vi "Hardware In - ECS - EPTx Interface.vi"(0 "FPGA 1 Ref":T2, 5 "FPGA 2 Ref":T2, 11 "FPGA Knock Ref":T2) -> (4 "EPT out":T3, 6 "Aux1Adv":sgl, 8 "Aux2Adv":sgl, 10 "Aux3Adv":sgl, 12 "Engine Status":T1, 13 "Knock.Intensity":sgl[](array[numeric]) format="%.6g", 14 "Knock.Results":bool[](array[boolean]), 15 "Aux4Adv":sgl)   [LabVIEW 2015, in "ECS-RT.lvlib"]
uses:
  ECS-RT.lvlib
  Typedefs/EPT/EPT Cluster.ctl
  <vilib>/Powertrain Controls/Device Drivers/Engine Position Tracking/EPTx/RevA/RT/Controls/EPTxData.ctl
  Typedefs/FPGA Refs/Generic FPGA Ref.ctl
  Typedefs/EPT/Engine Status.ctl
  <vilib>/Powertrain Controls/Device Drivers/Engine Position Tracking/EPTx/RevA/RT/Controls/EPTxState.ctl
  <vilib>/Powertrain Controls/Device Drivers/Engine Position Tracking/EPTx/RevA/RT/Controls/EPTxFilters.ctl
  <vilib>/Powertrain Controls/Device Drivers/Engine Position Tracking/EPTx/RevA/RT/Controls/Encoder Config.ctl
  <vilib>/Powertrain Controls/Device Drivers/FPGA Knock/RevA/RT/Controls/Knock Settings.ctl
  <vilib>/Powertrain Controls/Device Drivers/FPGA Knock/RevA/RT/Controls/Windows.ctl
  <vilib>/Utility/error.llb/Error Cluster From Error Code.vi
  <vilib>/rvi/errors/niLvFpgaAdjustHostInterfaceError.vi
  Globals/TDC Globals.vi
  <vilib>/rvi/interface/nirviReadWriteControl/nirviReadWriteControl.xnode
  NiFpgaLv.dll
  <vilib>/rvi/interface/Simulation/niFpgaSimulationCallBeginRW.vi
  ECS-Shared.lvlib
  <vilib>/Powertrain Controls/Device Drivers/Engine Position Tracking/EPTx/RevA/RT/EPTx - RevA - RT.lvlib
  <vilib>/Powertrain Controls/Device Drivers/FPGA Knock/RevA/RT/Knock - RevA - RT.lvlib
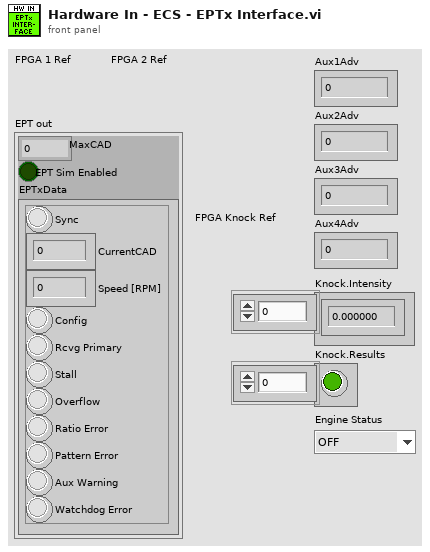
[diagram p1: front panel]
types:
  T1 = typedef "ECS-Shared.lvlib/Engine Status.ctl" = enum16{"OFF", "STALLED", "CRANKING", "RUNNING", "ACCEL", "DECEL", "SAFE"}
  T2 = typedef "ECS-Shared.lvlib/Generic FPGA Ref.ctl" = refnum<k20>
  T3 = typedef "ECS-Shared.lvlib/EPT Cluster.ctl" = cluster{"MaxCAD":sgl, "EPT Sim Enabled":bool, "EPTxData":T4}
  T4 = typedef "EPTx - RevA - RT.lvlib/EPTxData.ctl" = cluster{"Sync":bool, "CurrentCAD":sgl, "Speed [RPM]":sgl, "Config":bool, "Rcvg Primary":bool, "Stall":bool, "Overflow":bool, "Ratio Error":bool, "Pattern Error":bool, "Aux Warning":bool, "Watchdog Error":bool}
  T5 = enum8{"1 Sample/Pulse", "2 Sample/Pulse", "4 Sample/Pulse"}
  T6 = typedef "EPTx - RevA - RT.lvlib/Encoder Config.ctl" = cluster{"Tooth Count":u16, "Max Rate [Hz]":sgl, "Samples":enum8{"1 Sample/Pulse", "2 Sample/Pulse", "4 Sample/Pulse"}}
  T7 = typedef "EPTx - RevA - RT.lvlib/EPTxFilters.ctl" = cluster{"Primary [s]":sgl, "Aux 1 [s]":sgl, "Aux 2 [s]":sgl, "Aux 3 [s]":sgl, "Aux 4 [s]":sgl}
  T8 = typedef "EPTx - RevA - RT.lvlib/EPTxState.ctl" = cluster{"Sync Enable":bool, "Clear Errors":bool, "Sim Enable":bool, "Sim Speed [RPM]":sgl}
  T9 = typedef "Knock - RevA - RT.lvlib/Windows.ctl" = cluster{"Knock Start [CAD]":sgl, "Knock End [CAD]":sgl, "Reference End [CAD]":sgl, "Reference Start [CAD]":sgl}
  T10 = typedef "Knock - RevA - RT.lvlib/Knock Settings.ctl" = cluster{"Frequency [Hz]":sgl, "Low Cutoff [Hz]":sgl, "High Cutoff [Hz]":sgl, "Threshold":sgl}
  T11 = cluster{"Enable":bool, "RisingCAD":fxp<+,18,11>, "FallingCAD":fxp<+,18,11>}
  T12 = cluster{"Sync":bool, "CurrentCAD":fxp<+,18,11>, "MaxCAD":fxp<+,11,11>, "HistoryCAD":fxp<+,11,11>, "CADRate":fxp<+,22,8>, "AvgSpeed":fxp<+,17,15>, "Config":bool, "Rcvg Primary":bool, "Stall":bool, "Overflow":bool, "Ratio Error":bool, "Pattern Error":bool, "Aux Warning":bool, "Watchdog Error":bool}
  T13 = typedef "EPTx - RevA - RT.lvlib/EPTxSettings.ctl" = cluster{"Rotation":u8, "Ratios":sgl[], "Thresholds":sgl[], "Tooth":T14, "Pattern":T16[], "Token":T17[], "Aux Threshold Min":T20, "Aux Threshold Max":T20}
  T14 = typedef "EPTx - RevA - RT.lvlib/Settings - Tooth.ctl" = cluster{"Rising Edge":bool, "Falling Edge":bool, "Direction\nDetection":T15, "Level":bool, "Parameter":sgl}
  T15 = typedef "EPTx - RevA - RT.lvlib/Direction Detection.ctl" = enum16{"None", "Aux Signal", "Length"}
  T16 = typedef "EPTx - RevA - RT.lvlib/Settings - Pattern.ctl" = cluster{"Ratio Index":u8, "Ratio Count":u16, "Angle":sgl, "dAngle":sgl}
  T17 = typedef "EPTx - RevA - RT.lvlib/Settings - Token.ctl" = cluster{"Length":u16, "Start Index":u8, "Start Count":u16, "Aux 1":T18, "Aux 1 Type":T19, "Aux 1 Max":u16, "Aux 1 Min":u16, "Aux 2":T18, "Aux 2 Type":T19, "Aux 2 Max":u16, "Aux 2 Min":u16, "End Index":u8, "End Count":u16}
  T18 = typedef "EPTx - RevA - RT.lvlib/Aux Signal.ctl" = enum8{"---", "Aux 1", "Aux 2", "Aux 3", "Aux 4"}
  T19 = typedef "EPTx - RevA - RT.lvlib/Aux Type.ctl" = enum8{"Falling", "Rising", "Low", "High", "Ratio"}
  T20 = typedef "EPTx - RevA - RT.lvlib/Aux Threshold.ctl" = cluster{"Aux 1":sgl, "Aux 2":sgl, "Aux 3":sgl, "Aux 4":sgl}
  T21 = typedef "EPTx - RevA - FPGA.lvlib/EPTxConfig.ctl" = u64
  T22 = typedef "EPTx - RevA - FPGA.lvlib/EPTxControl.ctl" = cluster{"Sync Enable":bool, "Clear Errors":bool, "Sim Enable":bool, "Sim Rate":fxp<+,24,6>, "Watchdog":bool}
  T23 = typedef "Knock - RevA - FPGA.lvlib/Knock Settings.ctl" = cluster{"Threshold":fxp<+,8,4>, "Coeff A":fxp<+/-,16,4>[], "Coeff B":fxp<+/-,16,4>[]}
  T24 = typedef "Knock - RevA - FPGA.lvlib/EPTx Window.ctl" = cluster{"Knock Start":fxp<+,18,11>, "Knock End":fxp<+,18,11>, "Reference Start":fxp<+,18,11>, "Reference End":fxp<+,18,11>}
  T25 = typedef "EPTx - RevA - FPGA.lvlib/EPTxEncoderConfig.ctl" = cluster{"Tooth Count":fxp<+,12,12>, "Rate Limit":fxp<+,12,12>}
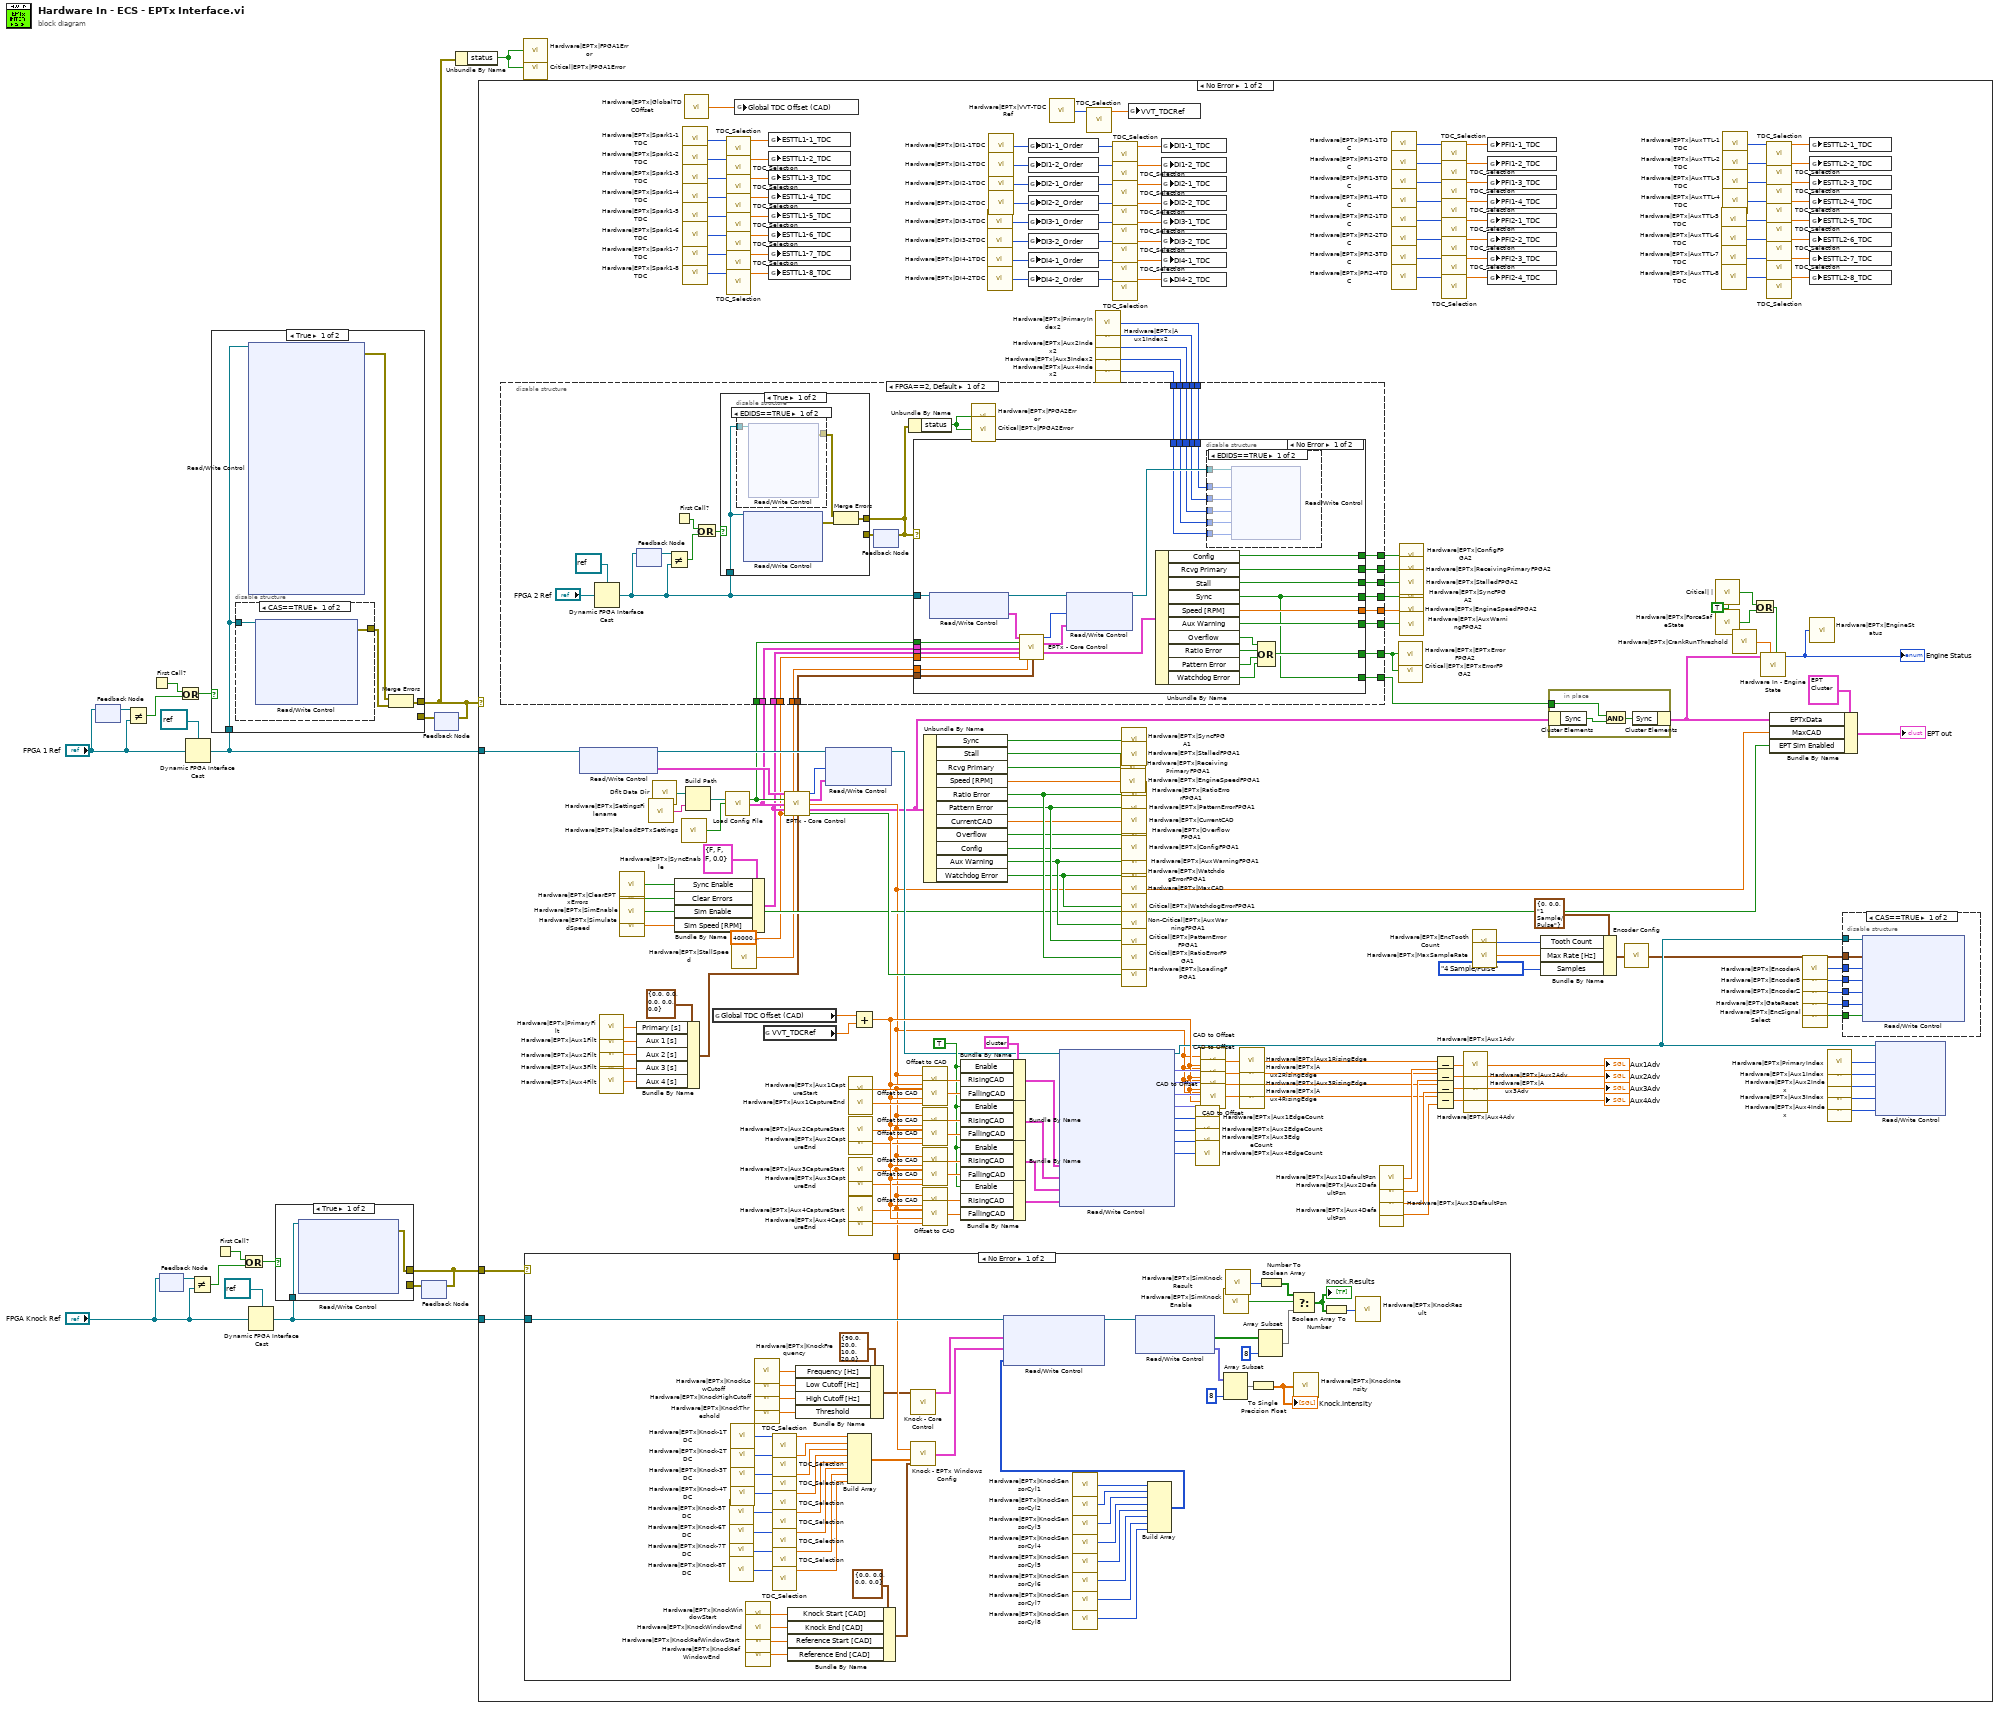
[diagram p0: block diagram]
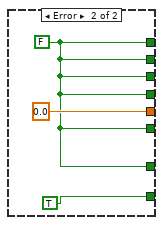
[diagram p6: hidden frame]
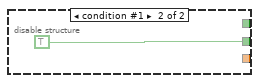
[diagram p9: hidden frame]
diagram:
  n1 = feedback #1() -> (w18:T2)  [unwired: 1 in]
  n2 = feedback-in #1("FPGA 1 Ref") -> ()
  n3 = Not Equal?(x=w18, y="FPGA 1 Ref") -> (x != y?=w19:bool)
  n4 = First Call?() -> (First Call?: T/F=w17:bool)
  n5 = feedback #2() -> (w8:T2)  [unwired: 1 in]
  n6 = feedback-in #2("FPGA Knock Ref") -> ()
  n7 = Or(x=w17, y=w19) -> (x .or. y?=w16:bool)
  n8 = Dynamic FPGA Interface Cast(Session In=refnum<k20> refnum ("EPT"), Type="FPGA 1 Ref") -> (Session Out=w12:refnum<k20>)
  n9 = Not Equal?(x=w8, y="FPGA Knock Ref") -> (x != y?=w9:bool)
  n10 = First Call?() -> (First Call?: T/F=w7:bool)
  n11 = Or(x=w7, y=w9) -> (x .or. y?=w6:bool)
  n12 = Dynamic FPGA Interface Cast(Session In=refnum<k20> refnum ("EPT"), Type="FPGA Knock Ref") -> (Session Out=w2:refnum<k20>)
  n13 = feedback #3() -> (w5:errorcluster)  [unwired: 1 in]
  n14 = case shown="True" w6 {
    tunnel: [w20 w22] -> w3
    tunnel: w5 -> [_ w22]
    tunnel: w2 -> [w21 _]
    frame True {
      n15 = xnode "Read/Write Control"("FPGA VI Reference In"=w21) -> ("error out"=w20:errorcluster)  [unwired: 4 in, 3 out]
    }
    frame False {
    }
  }
  n16 = feedback-in #3(w3) -> ()
  n17 = feedback #4() -> (w15:errorcluster)  [unwired: 1 in]
  n18 = case shown="True" w16 {
    tunnel: [w25 w29] -> w11
    tunnel: w15 -> [_ w29]
    tunnel: w12 -> [w26 _]
    frame True {
      n19 = disable-structure shown="CAS==TRUE" {
        disable-tunnel: w26 -> [w28 _]
        disable-tunnel: [w27 _] -> w23
        frame condition #0 (active) {
          n20 = xnode "Read/Write Control"("FPGA VI Reference In"=w28) -> ("error out"=w27:errorcluster)  [unwired: 7 in, 1 out]
        }
        frame condition #1 {
        }
      }
      n21 = xnode "Read/Write Control"("FPGA VI Reference In"=w26) -> ("error out"=w24:errorcluster)  [unwired: 12 in, 10 out]
      n22 = Merge Errors(w24, w23) -> (w25:errorcluster)
    }
    frame False {
    }
  }
  n23 = feedback-in #4(w11) -> ()
  n24 = Unbundle By Name(w11) -> ("status"=w10:bool)
  n25 = case shown="No Error" w11 {
    tunnel: w12 -> [w120 _]
    tunnel: w3 -> [w90 _]
    tunnel: w2 -> [w89 _]
    frame No Error {
      w109 = sgl 40000000.0 ("Frequency (40M) [Hz]")
      w125 = TRUE ("Enable")
      w147 = T11 {"Enable"=FALSE, "RisingCAD"=0.0, "FallingCAD"=0.0} ("EPTx.Aux1AngleCapture")
      n26 = xnode "Read/Write Control"("FPGA VI Reference In"=w120) -> ("FPGA VI Reference Out"=w190:refnum<k20>, "EPTxSupervisor"=w205:T12)  [unwired: 1 in, 1 out]
      n27 = call "Hardware|EPTx|PrimaryFilt"() -> ("Value"=w117:sgl)
      n28 = call "Hardware|EPTx|Aux1Filt"() -> ("Value"=w116:sgl)
      n29 = call "Hardware|EPTx|Aux2Filt"() -> ("Value"=w115:sgl)
      n30 = call "Hardware|EPTx|Aux3Filt"() -> ("Value"=w114:sgl)
      n31 = call "Hardware|EPTx|Aux4Filt"() -> ("Value"=w113:sgl)
      n32 = call "Hardware|EPTx|SyncEnable"() -> ("Value"=w122:bool)
      n33 = call "Hardware|EPTx|ClearEPTxErrors"() -> ("Value"=w101:bool)
      n34 = call "Hardware|EPTx|SimEnable"() -> ("Value"=w119:bool)
      n35 = call "Hardware|EPTx|SimulatedSpeed"() -> ("Value"=w121:sgl)
      n36 = Bundle By Name(cluster=T7 {"Primary [s]"=0.0, "Aux 1 [s]"=0.0, "Aux 2 [s]"=0.0, "Aux 3 [s]"=0.0, "Aux 4 [s]"=0.0} ("Filters (0)"), "Primary [s]"=w117, "Aux 1 [s]"=w116, "Aux 2 [s]"=w115, "Aux 3 [s]"=w114, "Aux 4 [s]"=w113) -> (w108:T7)
      n37 = call "Hardware|EPTx|SettingsFilename"() -> ("Value"=w186:string)
      n38 = call <vilib>:"Dflt Data Dir.vi"() -> ("App:Default Data Directory"=w187:path)
      n39 = Bundle By Name(cluster=T8 {"Sync Enable"=FALSE, "Clear Errors"=FALSE, "Sim Enable"=FALSE, "Sim Speed [RPM]"=0.0} ("EPTxState"), "Sync Enable"=w122, "Clear Errors"=w101, "Sim Enable"=w119, "Sim Speed [RPM]"=w121) -> (w110:T8)
      n40 = call "Hardware|EPTx|ReloadEPTxSettings"() -> ("Value"=w184:bool)
      n41 = call "Hardware|EPTx|Spark1-1TDC"() -> ("Value"=w76:u32)
      n42 = call "Hardware|EPTx|Spark1-2TDC"() -> ("Value"=w75:u32)
      n43 = call "Hardware|EPTx|Spark1-3TDC"() -> ("Value"=w74:u32)
      n44 = call "Hardware|EPTx|Spark1-4TDC"() -> ("Value"=w73:u32)
      n45 = call "Hardware|EPTx|Spark1-5TDC"() -> ("Value"=w72:u32)
      n46 = call "Hardware|EPTx|Spark1-6TDC"() -> ("Value"=w71:u32)
      n47 = call "Hardware|EPTx|Spark1-7TDC"() -> ("Value"=w70:u32)
      n48 = call "Hardware|EPTx|Spark1-8TDC"() -> ("Value"=w69:u32)
      n49 = call "Hardware|EPTx|GlobalTDCOffset"() -> ("Value"=w148:sgl)
      n50 = Build Path(base path=w187, name or relative path=w186) -> (appended path=w185:path)
      n51 = global read "TDC Globals.vi" "Global TDC Offset (CAD)"() -> (w214:sgl)
      n52 = call <vilib>:"Load Config File.vi"("Configuration Path"=w185, "Load"=w184) -> ("Loaded"=w112:bool, "EPTxSettings"=w111:T13)  [unwired: 12 in]
      n53 = call "TDC_Selection.vi"("TDC#"=w76) -> ("TDC"=w183:sgl)  [unwired: 10 in]
      n54 = call "TDC_Selection.vi"("TDC#"=w75) -> ("TDC"=w176:sgl)  [unwired: 10 in]
      n55 = call "TDC_Selection.vi"("TDC#"=w74) -> ("TDC"=w177:sgl)  [unwired: 10 in]
      n56 = call "TDC_Selection.vi"("TDC#"=w73) -> ("TDC"=w178:sgl)  [unwired: 10 in]
      n57 = call "TDC_Selection.vi"("TDC#"=w72) -> ("TDC"=w179:sgl)  [unwired: 10 in]
      n58 = call "TDC_Selection.vi"("TDC#"=w71) -> ("TDC"=w180:sgl)  [unwired: 10 in]
      n59 = call "TDC_Selection.vi"("TDC#"=w70) -> ("TDC"=w181:sgl)  [unwired: 10 in]
      n60 = call "TDC_Selection.vi"("TDC#"=w69) -> ("TDC"=w182:sgl)  [unwired: 10 in]
      n61 = call "Hardware|EPTx|StallSpeed"() -> ("Value"=w91:sgl)
      n62 = global write "TDC Globals.vi" "Global TDC Offset (CAD)"(w148) -> ()
      n63 = global read "TDC Globals.vi" "VVT_TDCRef"() -> (w99:sgl)
      n64 = global write "TDC Globals.vi" "ESTTL1-1_TDC"(w183) -> ()
      n65 = global write "TDC Globals.vi" "ESTTL1-2_TDC"(w176) -> ()
      n66 = global write "TDC Globals.vi" "ESTTL1-3_TDC"(w177) -> ()
      n67 = global write "TDC Globals.vi" "ESTTL1-4_TDC"(w178) -> ()
      n68 = global write "TDC Globals.vi" "ESTTL1-5_TDC"(w179) -> ()
      n69 = global write "TDC Globals.vi" "ESTTL1-6_TDC"(w180) -> ()
      n70 = global write "TDC Globals.vi" "ESTTL1-7_TDC"(w181) -> ()
      n71 = global write "TDC Globals.vi" "ESTTL1-8_TDC"(w182) -> ()
      n72 = call <vilib>:"EPTx - Core Control.vi"("EPTxSupervisor"=w205, "Load"=w112, "EPTxSettings"=w111, "EPTxState"=w110, "Frequency (40M) [Hz]"=w109, "Stall Speed (200) [RPM]"=w91, "Filters (0)"=w108) -> ("EPTxConfig"=w189:T21, "EPTxControl"=w188:T22, "Max CAD"=w88:sgl, "EPTxData"=w87:T4, "Loading"=w195:bool)  [unwired: 4 in]
      n73 = case shown="No Error" w90 {
        tunnel: w89 -> [w254 _]
        tunnel: w88 -> [w233 _]
        frame No Error {
          n74 = call "Hardware|EPTx|Knock-5TDC"() -> ("Value"=w267:u32)
          n75 = call "Hardware|EPTx|Knock-6TDC"() -> ("Value"=w266:u32)
          n76 = call "Hardware|EPTx|Knock-7TDC"() -> ("Value"=w265:u32)
          n77 = call "Hardware|EPTx|Knock-8TDC"() -> ("Value"=w264:u32)
          n78 = call "Hardware|EPTx|Knock-1TDC"() -> ("Value"=w271:u32)
          n79 = call "Hardware|EPTx|Knock-2TDC"() -> ("Value"=w270:u32)
          n80 = call "Hardware|EPTx|Knock-3TDC"() -> ("Value"=w269:u32)
          n81 = call "Hardware|EPTx|Knock-4TDC"() -> ("Value"=w268:u32)
          n82 = call "Hardware|EPTx|KnockWindowStart"() -> ("Value"=w275:sgl)
          n83 = call "Hardware|EPTx|KnockWindowEnd"() -> ("Value"=w274:sgl)
          n84 = call "Hardware|EPTx|KnockRefWindowStart"() -> ("Value"=w273:sgl)
          n85 = call "Hardware|EPTx|KnockRefWindowEnd"() -> ("Value"=w272:sgl)
          n86 = call "Hardware|EPTx|KnockFrequency"() -> ("Value"=w279:sgl)
          n87 = call "Hardware|EPTx|KnockLowCutoff"() -> ("Value"=w278:sgl)
          n88 = call "Hardware|EPTx|KnockHighCutoff"() -> ("Value"=w277:sgl)
          n89 = call "Hardware|EPTx|KnockThreshold"() -> ("Value"=w276:sgl)
          n90 = call "TDC_Selection.vi"("TDC#"=w271) -> ("TDC"=w263:sgl)  [unwired: 10 in]
          n91 = call "TDC_Selection.vi"("TDC#"=w270) -> ("TDC"=w262:sgl)  [unwired: 10 in]
          n92 = call "TDC_Selection.vi"("TDC#"=w269) -> ("TDC"=w261:sgl)  [unwired: 10 in]
          n93 = call "TDC_Selection.vi"("TDC#"=w268) -> ("TDC"=w260:sgl)  [unwired: 10 in]
          n94 = call "TDC_Selection.vi"("TDC#"=w267) -> ("TDC"=w259:sgl)  [unwired: 10 in]
          n95 = call "TDC_Selection.vi"("TDC#"=w266) -> ("TDC"=w258:sgl)  [unwired: 10 in]
          n96 = call "TDC_Selection.vi"("TDC#"=w265) -> ("TDC"=w257:sgl)  [unwired: 10 in]
          n97 = call "TDC_Selection.vi"("TDC#"=w264) -> ("TDC"=w256:sgl)  [unwired: 10 in]
          n98 = Bundle By Name(cluster=T9 {"Knock Start [CAD]"=0.0, "Knock End [CAD]"=0.0, "Reference End [CAD]"=0.0, "Reference Start [CAD]"=0.0} ("Windows"), "Knock Start [CAD]"=w275, "Knock End [CAD]"=w274, "Reference Start [CAD]"=w273, "Reference End [CAD]"=w272) -> (w234:T9)
          n99 = Bundle By Name(cluster=T10 {"Frequency [Hz]"=90.0, "Low Cutoff [Hz]"=20.0, "High Cutoff [Hz]"=10.0, "Threshold"=20.0} ("Knock Settings"), "Frequency [Hz]"=w279, "Low Cutoff [Hz]"=w278, "High Cutoff [Hz]"=w277, "Threshold"=w276) -> (w232:T10)
          n100 = Build Array(w263, w262, w261, w260, w259, w258, w257, w256) -> (w255:sgl[])
          n101 = call <vilib>:"Knock - Core Control.vi"("Knock Settings"=w232) -> ("Knock Settings"=w280:T23)  [unwired: 13 in, 1 out]
          n102 = call <vilib>:"Knock - EPTx Windows Config.vi"("Max CAD"=w233, "Cylinder Offset [CAD]"=w255, "Windows"=w234) -> ("EPTx Windows"=w281:cluster{"Index":fxp<+,4,4>, "EPT Windows":T24})  [unwired: 12 in]
          n103 = call "Hardware|EPTx|KnockSensorCyl1"() -> ("Value"=w245:u32)
          n104 = call "Hardware|EPTx|KnockSensorCyl2"() -> ("Value"=w244:u32)
          n105 = call "Hardware|EPTx|KnockSensorCyl3"() -> ("Value"=w243:u32)
          n106 = call "Hardware|EPTx|KnockSensorCyl4"() -> ("Value"=w242:u32)
          n107 = call "Hardware|EPTx|KnockSensorCyl5"() -> ("Value"=w241:u32)
          n108 = call "Hardware|EPTx|KnockSensorCyl6"() -> ("Value"=w240:u32)
          n109 = call "Hardware|EPTx|KnockSensorCyl7"() -> ("Value"=w239:u32)
          n110 = call "Hardware|EPTx|KnockSensorCyl8"() -> ("Value"=w238:u32)
          n111 = Build Array(w245, w244, w243, w242, w241, w240, w239, w238) -> (w237:u32[])
          n112 = xnode "Read/Write Control"("FPGA VI Reference In"=w254, "Knock.Settings"=w280, "Knock.Windows"=w281, "Knock.SensorIndices"=w237) -> ("FPGA VI Reference Out"=w253:refnum<k20>)  [unwired: 1 in, 1 out]
          n113 = xnode "Read/Write Control"("FPGA VI Reference In"=w253) -> ("Knock.Results"=w246:bool[], "Knock.Intensity"=w252:fxp<+,8,4>[])  [unwired: 1 in, 2 out]
          n114 = Array Subset(array=w252, length=8) -> (w250:fxp<+,8,4>[])  [unwired: 1 in]
          n115 = call "Hardware|EPTx|SimKnockEnable"() -> ("Value"=w231:bool)
          n116 = call "Hardware|EPTx|SimKnockResult"() -> ("Value"=w228:u8)
          n117 = To Single Precision Float(number=w250) -> (single precision float=w248:sgl[])
          "Knock.Intensity" <- w248
          n118 = Array Subset(array=w246, length=8) -> (w230:bool[])  [unwired: 1 in]
          n119 = Number To Boolean Array(number=w228) -> (Boolean array=w227:bool[])
          n120 = Select(t=w227, s=w231, f=w230) -> (s? t:f=w229:bool[])
          "Knock.Results" <- w229
          n121 = call "Hardware|EPTx|KnockIntensity"("Value"=w248) -> ()
          n122 = Boolean Array To Number(Boolean array=w229) -> (number=w249:u32)
          n123 = call "Hardware|EPTx|KnockResult"("Value"=w249) -> ()
        }
        frame Error {
        }
      }
      n124 = xnode "Read/Write Control"("FPGA VI Reference In"=w190, "EPTxConfig"=w189, "EPTxControl"=w188) -> ("FPGA VI Reference Out"=w123:refnum<k20>)  [unwired: 1 in, 1 out]
      n125 = call "Hardware|EPTx|Aux1CaptureStart"() -> ("Value"=w133:sgl)
      n126 = call "Hardware|EPTx|Aux1CaptureEnd"() -> ("Value"=w134:sgl)
      n127 = call "Hardware|EPTx|Aux2CaptureStart"() -> ("Value"=w130:sgl)
      n128 = call "Hardware|EPTx|Aux2CaptureEnd"() -> ("Value"=w131:sgl)
      n129 = call "Hardware|EPTx|Aux3CaptureStart"() -> ("Value"=w129:sgl)
      n130 = call "Hardware|EPTx|Aux3CaptureEnd"() -> ("Value"=w128:sgl)
      n131 = call "Hardware|EPTx|Aux4CaptureStart"() -> ("Value"=w127:sgl)
      n132 = call "Hardware|EPTx|Aux4CaptureEnd"() -> ("Value"=w126:sgl)
      n133 = Add(x=w214, y=w99) -> (x+y=w132:sgl)
      n134 = call <vilib>:"Offset to CAD.vi"("Max CAD"=w88, "Cylinder TDC [Absolute CAD]"=w132, "Offset [DBTDC]"=w133) -> ("CAD [Absolute CAD]"=w142:sgl)  [unwired: 12 in]
      n135 = call <vilib>:"Offset to CAD.vi"("Max CAD"=w88, "Cylinder TDC [Absolute CAD]"=w132, "Offset [DBTDC]"=w134) -> ("CAD [Absolute CAD]"=w141:sgl)  [unwired: 12 in]
      n136 = call <vilib>:"Offset to CAD.vi"("Max CAD"=w88, "Cylinder TDC [Absolute CAD]"=w132, "Offset [DBTDC]"=w130) -> ("CAD [Absolute CAD]"=w140:sgl)  [unwired: 12 in]
      n137 = call <vilib>:"Offset to CAD.vi"("Max CAD"=w88, "Cylinder TDC [Absolute CAD]"=w132, "Offset [DBTDC]"=w131) -> ("CAD [Absolute CAD]"=w139:sgl)  [unwired: 12 in]
      n138 = call <vilib>:"Offset to CAD.vi"("Max CAD"=w88, "Cylinder TDC [Absolute CAD]"=w132, "Offset [DBTDC]"=w129) -> ("CAD [Absolute CAD]"=w138:sgl)  [unwired: 12 in]
      n139 = call <vilib>:"Offset to CAD.vi"("Max CAD"=w88, "Cylinder TDC [Absolute CAD]"=w132, "Offset [DBTDC]"=w128) -> ("CAD [Absolute CAD]"=w135:sgl)  [unwired: 12 in]
      n140 = call <vilib>:"Offset to CAD.vi"("Max CAD"=w88, "Cylinder TDC [Absolute CAD]"=w132, "Offset [DBTDC]"=w127) -> ("CAD [Absolute CAD]"=w137:sgl)  [unwired: 12 in]
      n141 = call <vilib>:"Offset to CAD.vi"("Max CAD"=w88, "Cylinder TDC [Absolute CAD]"=w132, "Offset [DBTDC]"=w126) -> ("CAD [Absolute CAD]"=w136:sgl)  [unwired: 12 in]
      n142 = Unbundle By Name(w87) -> ("Sync"=w204:bool, "Stall"=w203:bool, "Rcvg Primary"=w107:bool, "Speed [RPM]"=w92:sgl, "Ratio Error"=w202:bool, "Pattern Error"=w201:bool, "CurrentCAD"=w200:sgl, "Overflow"=w197:bool, "Config"=w196:bool, "Aux Warning"=w199:bool, "Watchdog Error"=w198:bool)
      n143 = Bundle By Name(cluster=w147, "Enable"=w125, "RisingCAD"=w142, "FallingCAD"=w141) -> (w146:T11)
      n144 = Bundle By Name(cluster=w147, "Enable"=w125, "RisingCAD"=w140, "FallingCAD"=w139) -> (w145:T11)
      n145 = Bundle By Name(cluster=w147, "Enable"=w125, "RisingCAD"=w138, "FallingCAD"=w135) -> (w144:T11)
      n146 = Bundle By Name(cluster=w147, "Enable"=w125, "RisingCAD"=w137, "FallingCAD"=w136) -> (w143:T11)
      n147 = call "Hardware|EPTx|DI3-1TDC"() -> ("Value"=w155:u32)
      n148 = call "Hardware|EPTx|DI3-2TDC"() -> ("Value"=w154:u32)
      n149 = call "Hardware|EPTx|DI4-1TDC"() -> ("Value"=w78:u32)
      n150 = call "Hardware|EPTx|DI4-2TDC"() -> ("Value"=w77:u32)
      n151 = call "Hardware|EPTx|DI1-1TDC"() -> ("Value"=w159:u32)
      n152 = call "Hardware|EPTx|DI1-2TDC"() -> ("Value"=w158:u32)
      n153 = call "Hardware|EPTx|DI2-1TDC"() -> ("Value"=w157:u32)
      n154 = call "Hardware|EPTx|DI2-2TDC"() -> ("Value"=w156:u32)
      n155 = global write "TDC Globals.vi" "DI1-1_Order"(w159) -> ()
      n156 = global write "TDC Globals.vi" "DI1-2_Order"(w158) -> ()
      n157 = global write "TDC Globals.vi" "DI2-1_Order"(w157) -> ()
      n158 = global write "TDC Globals.vi" "DI2-2_Order"(w156) -> ()
      n159 = global write "TDC Globals.vi" "DI3-1_Order"(w155) -> ()
      n160 = global write "TDC Globals.vi" "DI3-2_Order"(w154) -> ()
      n161 = global write "TDC Globals.vi" "DI4-1_Order"(w78) -> ()
      n162 = global write "TDC Globals.vi" "DI4-2_Order"(w77) -> ()
      n163 = call "Hardware|EPTx|VVT-TDCRef"() -> ("Value"=w149:u32)
      n164 = xnode "Read/Write Control"("FPGA VI Reference In"=w123, "EPTx.Aux1AngleCapture"=w146, "EPTx.Aux2AngleCapture"=w145, "EPTx.Aux3AngleCapture"=w144, "EPTx.Aux4AngleCapture"=w143) -> ("FPGA VI Reference Out"=w98:refnum<k20>, "EPTx.Aux1CaptureCAD"=w218:fxp<+,18,11>, "EPTx.Aux2CaptureCAD"=w217:fxp<+,18,11>, "EPTx.Aux3CaptureCAD"=w216:fxp<+,18,11>, "EPTx.Aux4CaptureCAD"=w215:fxp<+,18,11>, "EPTx.Aux1EdgeCount"=w194:u8, "EPTx.Aux2EdgeCount"=w193:u8, "EPTx.Aux3EdgeCount"=w192:u8, "EPTx.Aux4EdgeCount"=w191:u8)  [unwired: 1 in, 1 out]
      n165 = call "TDC_Selection.vi"("TDC#"=w149) -> ("TDC"=w100:sgl)  [unwired: 10 in]
      n166 = call "Hardware|EPTx|PrimaryIndex2"() -> ("Value"=w36:u8)
      n167 = call "Hardware|EPTx|Aux1Index2"() -> ("Value"=w35:u8)
      n168 = call "Hardware|EPTx|Aux2Index2"() -> ("Value"=w34:u8)
      n169 = call "Hardware|EPTx|Aux3Index2"() -> ("Value"=w33:u8)
      n170 = call "Hardware|EPTx|Aux4Index2"() -> ("Value"=w32:u8)
      n171 = disable-structure shown="FPGA==2, Default" {
        disable-tunnel: [w311 TRUE] -> w30
        disable-tunnel: w112 -> [w309 _]
        disable-tunnel: w111 -> [w308 _]
        disable-tunnel: w110 -> [w307 _]
        disable-tunnel: w109 -> [w306 _]
        disable-tunnel: w91 -> [w305 _]
        disable-tunnel: w108 -> [w304 _]
        disable-tunnel: [w300 _] -> w42
        disable-tunnel: [w299 _] -> w41
        disable-tunnel: [w298 _] -> w40
        disable-tunnel: [w297 _] -> w39
        disable-tunnel: [w296 _] -> w38
        disable-tunnel: [w295 _] -> w37
        disable-tunnel: w36 -> [w294 _]
        disable-tunnel: w35 -> [w293 _]
        disable-tunnel: w34 -> [w292 _]
        disable-tunnel: w33 -> [w291 _]
        disable-tunnel: w32 -> [w290 _]
        disable-tunnel: [w289 _] -> w31
        frame condition #0 (active) {
          n172 = Dynamic FPGA Interface Cast(Session In=refnum<k20> refnum ("EPT"), Type="FPGA 2 Ref") -> (Session Out=w313:refnum<k20>)
          n173 = feedback #5() -> (w317:refnum<k20>)  [unwired: 1 in]
          n174 = feedback-in #5(w313) -> ()
          n175 = Not Equal?(x=w317, y=w313) -> (x != y?=w315:bool)
          n176 = First Call?() -> (First Call?: T/F=w316:bool)
          n177 = Or(x=w316, y=w315) -> (x .or. y?=w314:bool)
          n178 = feedback #6() -> (w312:errorcluster)  [unwired: 1 in]
          n179 = case shown="True" w314 {
            tunnel: w313 -> [w359 _]
            tunnel: w312 -> [_ w362]
            tunnel: [w356 w362] -> w301
            frame True {
              n180 = disable-structure shown="EDIDS==TRUE" {
                disable-tunnel: w359 -> [w361 _]
                disable-tunnel: [w360 _] -> w357
                frame condition #0 {
                  n181 = xnode "Read/Write Control"("FPGA VI Reference In"=w361) -> ("error out"=w360:errorcluster)  [unwired: 6 in, 1 out]
                }
                frame condition #1 (active) {
                }
              }
              n182 = xnode "Read/Write Control"("FPGA VI Reference In"=w359) -> ("error out"=w358:errorcluster)  [unwired: 3 in, 2 out]
              n183 = Merge Errors(w357, w358) -> (w356:errorcluster)
            }
            frame False {
            }
          }
          n184 = feedback-in #6(w301) -> ()
          n185 = Unbundle By Name(w301) -> ("status"=w303:bool)
          n186 = case shown="No Error" w301 {
            tunnel: w313 -> [w346 _]
            tunnel: [w323 w354] -> w311
            tunnel: w309 -> [w344 _]
            tunnel: w308 -> [w343 _]
            tunnel: w307 -> [w342 _]
            tunnel: w306 -> [w341 _]
            tunnel: w305 -> [w340 _]
            tunnel: w304 -> [w339 _]
            tunnel: [w333 w354] -> w300
            tunnel: [w332 w354] -> w299
            tunnel: [w331 w354] -> w298
            tunnel: [w330 sgl 0.0 ("Speed [RPM]")] -> w297
            tunnel: [w329 w354] -> w296
            tunnel: [w324 w354] -> w295
            tunnel: w294 -> [w322 _]
            tunnel: w293 -> [w321 _]
            tunnel: w292 -> [w320 _]
            tunnel: w291 -> [w319 _]
            tunnel: w290 -> [w318 _]
            tunnel: [w323 TRUE ("Sync")] -> w289
            frame No Error {
              n187 = xnode "Read/Write Control"("FPGA VI Reference In"=w346) -> ("FPGA VI Reference Out"=w337:refnum<k20>, "EPTxSupervisor"=w345:T12)  [unwired: 1 in, 1 out]
              n188 = call <vilib>:"EPTx - Core Control.vi"("EPTxSupervisor"=w345, "Load"=w344, "EPTxSettings"=w343, "EPTxState"=w342, "Frequency (40M) [Hz]"=w341, "Stall Speed (200) [RPM]"=w340, "Filters (0)"=w339) -> ("EPTxConfig"=w336:T21, "EPTxControl"=w335:T22, "EPTxData"=w338:T4)  [unwired: 4 in, 2 out]
              n189 = xnode "Read/Write Control"("FPGA VI Reference In"=w337, "EPTxConfig"=w336, "EPTxControl"=w335) -> ("FPGA VI Reference Out"=w334:refnum<k20>)  [unwired: 1 in, 1 out]
              n190 = Unbundle By Name(w338) -> ("Config"=w333:bool, "Rcvg Primary"=w332:bool, "Stall"=w331:bool, "Sync"=w323:bool, "Speed [RPM]"=w330:sgl, "Aux Warning"=w329:bool, "Overflow"=w328:bool, "Ratio Error"=w327:bool, "Pattern Error"=w326:bool, "Watchdog Error"=w325:bool)
              n191 = disable-structure shown="EDIDS==TRUE" {
                disable-tunnel: w334 -> [w352 _]
                disable-tunnel: w322 -> [w351 _]
                disable-tunnel: w321 -> [w350 _]
                disable-tunnel: w320 -> [w349 _]
                disable-tunnel: w319 -> [w348 _]
                disable-tunnel: w318 -> [w347 _]
                frame condition #0 {
                  n192 = xnode "Read/Write Control"("FPGA VI Reference In"=w352, "EPTx.Primary"=w351, "EPTx.Aux1"=w350, "EPTx.Aux2"=w349, "EPTx.Aux3"=w348, "EPTx.Aux4"=w347) -> ()  [unwired: 1 in, 2 out]
                }
                frame condition #1 (active) {
                }
              }
              n193 = Compound Arithmetic op=OR(w328, w327, w326, w325) -> (w324:bool)
            }
            frame Error {
              w354 = FALSE ("Stall")
            }
          }
          n194 = call "Hardware|EPTx|FPGA2Error"("Value"=w303) -> ()
          n195 = call "Critical|EPTx|FPGA2Error"("Fault"=w303) -> ()  [unwired: 2 in]
        }
        frame condition #1 {
        }
      }
      n196 = call "TDC_Selection.vi"("TDC#"=w159) -> ("TDC"=w175:sgl)  [unwired: 10 in]
      n197 = call "TDC_Selection.vi"("TDC#"=w158) -> ("TDC"=w174:sgl)  [unwired: 10 in]
      n198 = call "TDC_Selection.vi"("TDC#"=w157) -> ("TDC"=w173:sgl)  [unwired: 10 in]
      n199 = call "TDC_Selection.vi"("TDC#"=w156) -> ("TDC"=w172:sgl)  [unwired: 10 in]
      n200 = call "TDC_Selection.vi"("TDC#"=w155) -> ("TDC"=w171:sgl)  [unwired: 10 in]
      n201 = call "TDC_Selection.vi"("TDC#"=w154) -> ("TDC"=w170:sgl)  [unwired: 10 in]
      n202 = call "TDC_Selection.vi"("TDC#"=w78) -> ("TDC"=w169:sgl)  [unwired: 10 in]
      n203 = call "TDC_Selection.vi"("TDC#"=w77) -> ("TDC"=w168:sgl)  [unwired: 10 in]
      n204 = call "Hardware|EPTx|ReceivingPrimaryFPGA1"("Value"=w107) -> ()
      n205 = call "Hardware|EPTx|EngineSpeedFPGA1"("Value"=w92) -> ()
      n206 = call "Hardware|EPTx|SyncFPGA1"("Value"=w204) -> ()
      n207 = call "Hardware|EPTx|StalledFPGA1"("Value"=w203) -> ()
      n208 = call "Hardware|EPTx|RatioErrorFPGA1"("Value"=w202) -> ()
      n209 = call "Hardware|EPTx|PatternErrorFPGA1"("Value"=w201) -> ()
      n210 = call "Hardware|EPTx|CurrentCAD"("Value"=w200) -> ()
      n211 = call "Hardware|EPTx|OverflowFPGA1"("Value"=w197) -> ()
      n212 = call "Hardware|EPTx|ConfigFPGA1"("Value"=w196) -> ()
      n213 = call "Hardware|EPTx|AuxWarningFPGA1"("Value"=w199) -> ()
      n214 = call "Hardware|EPTx|WatchdogErrorFPGA1"("Value"=w198) -> ()
      n215 = call "Hardware|EPTx|MaxCAD"("Value"=w88) -> ()
      n216 = call "Critical|EPTx|WatchdogErrorFPGA1"("Fault"=w198) -> ()  [unwired: 2 in]
      n217 = call "Non-Critical|EPTx|AuxWarningFPGA1"("Fault"=w199) -> ()  [unwired: 2 in]
      n218 = call "Critical|EPTx|PatternErrorFPGA1"("Fault"=w201) -> ()  [unwired: 2 in]
      n219 = call "Critical|EPTx|RatioErrorFPGA1"("Fault"=w202) -> ()  [unwired: 2 in]
      n220 = call "Hardware|EPTx|LoadingFPGA1"("Value"=w195) -> ()
      n221 = global write "TDC Globals.vi" "VVT_TDCRef"(w100) -> ()
      n222 = global write "TDC Globals.vi" "DI1-1_TDC"(w175) -> ()
      n223 = global write "TDC Globals.vi" "DI1-2_TDC"(w174) -> ()
      n224 = global write "TDC Globals.vi" "DI2-1_TDC"(w173) -> ()
      n225 = global write "TDC Globals.vi" "DI2-2_TDC"(w172) -> ()
      n226 = global write "TDC Globals.vi" "DI3-1_TDC"(w171) -> ()
      n227 = global write "TDC Globals.vi" "DI3-2_TDC"(w170) -> ()
      n228 = global write "TDC Globals.vi" "DI4-1_TDC"(w169) -> ()
      n229 = global write "TDC Globals.vi" "DI4-2_TDC"(w168) -> ()
      n230 = call "Hardware|EPTx|Aux1EdgeCount"("Value"=w194) -> ()
      n231 = call "Hardware|EPTx|Aux2EdgeCount"("Value"=w193) -> ()
      n232 = call "Hardware|EPTx|Aux3EdgeCount"("Value"=w192) -> ()
      n233 = call "Hardware|EPTx|Aux4EdgeCount"("Value"=w191) -> ()
      n234 = call <vilib>:"CAD to Offset.vi"("Max CAD"=w88, "Cylinder TDC [Absolute CAD]"=w132, "CAD [Absolute CAD]"=w218) -> ("Offset [DBTDC]"=w213:sgl)  [unwired: 12 in]
      n235 = call <vilib>:"CAD to Offset.vi"("Max CAD"=w88, "Cylinder TDC [Absolute CAD]"=w132, "CAD [Absolute CAD]"=w217) -> ("Offset [DBTDC]"=w212:sgl)  [unwired: 12 in]
      n236 = call <vilib>:"CAD to Offset.vi"("Max CAD"=w88, "Cylinder TDC [Absolute CAD]"=w132, "CAD [Absolute CAD]"=w216) -> ("Offset [DBTDC]"=w209:sgl)  [unwired: 12 in]
      n237 = call <vilib>:"CAD to Offset.vi"("Max CAD"=w88, "Cylinder TDC [Absolute CAD]"=w132, "CAD [Absolute CAD]"=w215) -> ("Offset [DBTDC]"=w206:sgl)  [unwired: 12 in]
      n238 = call "Hardware|EPTx|Aux1RisingEdge"("Value"=w213) -> ()
      n239 = call "Hardware|EPTx|Aux2RisingEdge"("Value"=w212) -> ()
      n240 = call "Hardware|EPTx|Aux3RisingEdge"("Value"=w209) -> ()
      n241 = call "Hardware|EPTx|Aux4RisingEdge"("Value"=w206) -> ()
      n242 = call "Hardware|EPTx|Aux1DefaultPsn"() -> ("Value"=w222:sgl)
      n243 = call "Hardware|EPTx|Aux2DefaultPsn"() -> ("Value"=w223:sgl)
      n244 = call "Hardware|EPTx|Aux3DefaultPsn"() -> ("Value"=w208:sgl)
      n245 = call "Hardware|EPTx|Aux4DefaultPsn"() -> ("Value"=w207:sgl)
      n246 = call "Hardware|EPTx|PFI1-1TDC"() -> ("Value"=w153:u32)
      n247 = call "Hardware|EPTx|PFI1-2TDC"() -> ("Value"=w152:u32)
      n248 = call "Hardware|EPTx|PFI1-3TDC"() -> ("Value"=w151:u32)
      n249 = call "Hardware|EPTx|PFI1-4TDC"() -> ("Value"=w150:u32)
      n250 = call "Hardware|EPTx|PFI2-1TDC"() -> ("Value"=w68:u32)
      n251 = call "Hardware|EPTx|PFI2-2TDC"() -> ("Value"=w67:u32)
      n252 = call "Hardware|EPTx|PFI2-3TDC"() -> ("Value"=w66:u32)
      n253 = call "Hardware|EPTx|PFI2-4TDC"() -> ("Value"=w65:u32)
      n254 = call "Hardware|EPTx|EPTxErrorFPGA2"("Value"=w37) -> ()
      n255 = call "Critical|EPTx|EPTxErrorFPGA2"("Fault"=w37) -> ()  [unwired: 2 in]
      n256 = call "Hardware|EPTx|ConfigFPGA2"("Value"=w42) -> ()
      n257 = call "Hardware|EPTx|ReceivingPrimaryFPGA2"("Value"=w41) -> ()
      n258 = call "Hardware|EPTx|StalledFPGA2"("Value"=w40) -> ()
      n259 = call "Hardware|EPTx|SyncFPGA2"("Value"=w30) -> ()
      n260 = call "Hardware|EPTx|EngineSpeedFPGA2"("Value"=w39) -> ()
      n261 = call "Hardware|EPTx|AuxWarningFPGA2"("Value"=w38) -> ()
      n262 = Subtract(x=w213, y=w222) -> (x-y=w220:sgl)
      "Aux1Adv" <- w220
      n263 = Subtract(x=w212, y=w223) -> (x-y=w219:sgl)
      "Aux2Adv" <- w219
      n264 = Subtract(x=w209, y=w208) -> (x-y=w210:sgl)
      "Aux3Adv" <- w210
      n265 = Subtract(x=w206, y=w207) -> (x-y=w211:sgl)
      "Aux4Adv" <- w211
      n266 = call "TDC_Selection.vi"("TDC#"=w153) -> ("TDC"=w166:sgl)  [unwired: 10 in]
      n267 = call "TDC_Selection.vi"("TDC#"=w152) -> ("TDC"=w165:sgl)  [unwired: 10 in]
      n268 = call "TDC_Selection.vi"("TDC#"=w151) -> ("TDC"=w164:sgl)  [unwired: 10 in]
      n269 = call "TDC_Selection.vi"("TDC#"=w150) -> ("TDC"=w163:sgl)  [unwired: 10 in]
      n270 = call "TDC_Selection.vi"("TDC#"=w68) -> ("TDC"=w162:sgl)  [unwired: 10 in]
      n271 = call "TDC_Selection.vi"("TDC#"=w67) -> ("TDC"=w161:sgl)  [unwired: 10 in]
      n272 = call "TDC_Selection.vi"("TDC#"=w66) -> ("TDC"=w160:sgl)  [unwired: 10 in]
      n273 = call "TDC_Selection.vi"("TDC#"=w65) -> ("TDC"=w167:sgl)  [unwired: 10 in]
      n274 = call "Hardware|EPTx|Aux1Adv"("Value"=w220) -> ()
      n275 = call "Hardware|EPTx|Aux2Adv"("Value"=w219) -> ()
      n276 = call "Hardware|EPTx|Aux3Adv"("Value"=w210) -> ()
      n277 = call "Hardware|EPTx|Aux4Adv"("Value"=w211) -> ()
      n278 = call "Hardware|EPTx|EncToothCount"() -> ("Value"=w60:u32)
      n279 = call "Hardware|EPTx|MaxSampleRate"() -> ("Value"=w61:sgl)
      n280 = global write "TDC Globals.vi" "PFI1-1_TDC"(w166) -> ()
      n281 = global write "TDC Globals.vi" "PFI1-2_TDC"(w165) -> ()
      n282 = global write "TDC Globals.vi" "PFI1-3_TDC"(w164) -> ()
      n283 = global write "TDC Globals.vi" "PFI1-4_TDC"(w163) -> ()
      n284 = global write "TDC Globals.vi" "PFI2-1_TDC"(w162) -> ()
      n285 = global write "TDC Globals.vi" "PFI2-2_TDC"(w161) -> ()
      n286 = global write "TDC Globals.vi" "PFI2-3_TDC"(w160) -> ()
      n287 = global write "TDC Globals.vi" "PFI2-4_TDC"(w167) -> ()
      n288 = Bundle By Name(cluster=T6 {"Tooth Count"=0, "Max Rate [Hz]"=0.0, "Samples"=enum."1 Sample/Pulse"} ("EncoderConfig"), "Tooth Count"=w60, "Max Rate [Hz]"=w61, "Samples"=T5."4 Sample/Pulse") -> (w62:T6)
      n289 = in-place {
        in-place-border: w31 -> [w225]
        n290 = in-place-cluster #7(w87) -> ("Sync"=w226:bool)
        n291 = And(x=w225, y=w226) -> (x .and. y?=w224:bool)
        n292 = in-place-cluster #7("Sync"=w224) -> (w85:T4)
      }
      n293 = call <vilib>:"Encoder Config.vi"("EncoderConfig"=w62) -> ("EPTxEncoderConfig"=w64:T25)  [unwired: 14 in]
      n294 = call "Critical| |"("UnAcknowledged (F)"=TRUE) -> ("Fault"=w83:bool)  [unwired: 1 in]
      n295 = call "Hardware|EPTx|ForceSafeState"() -> ("Value"=w82:bool)
      n296 = call "Hardware|EPTx|AuxTTL-5TDC"() -> ("Value"=w54:u32)
      n297 = call "Hardware|EPTx|AuxTTL-6TDC"() -> ("Value"=w53:u32)
      n298 = call "Hardware|EPTx|AuxTTL-7TDC"() -> ("Value"=w52:u32)
      n299 = call "Hardware|EPTx|AuxTTL-8TDC"() -> ("Value"=w51:u32)
      n300 = call "Hardware|EPTx|AuxTTL-1TDC"() -> ("Value"=w58:u32)
      n301 = call "Hardware|EPTx|AuxTTL-2TDC"() -> ("Value"=w57:u32)
      n302 = call "Hardware|EPTx|AuxTTL-3TDC"() -> ("Value"=w56:u32)
      n303 = call "Hardware|EPTx|AuxTTL-4TDC"() -> ("Value"=w55:u32)
      n304 = call "Hardware|EPTx|CrankRunThreshold"() -> ("Value"=w80:sgl)
      n305 = Or(x=w83, y=w82) -> (x .or. y?=w81:bool)
      n306 = call "Hardware In - Engine State.vi"("Set Safe State"=w81, "CrankRanThreshold"=w80, "EPTxData"=w85) -> ("Engine Status"=w79:T1)  [unwired: 8 in]
      "Engine Status" <- w79
      n307 = call "TDC_Selection.vi"("TDC#"=w58) -> ("TDC"=w43:sgl)  [unwired: 10 in]
      n308 = call "TDC_Selection.vi"("TDC#"=w57) -> ("TDC"=w50:sgl)  [unwired: 10 in]
      n309 = call "TDC_Selection.vi"("TDC#"=w56) -> ("TDC"=w49:sgl)  [unwired: 10 in]
      n310 = call "TDC_Selection.vi"("TDC#"=w55) -> ("TDC"=w48:sgl)  [unwired: 10 in]
      n311 = call "TDC_Selection.vi"("TDC#"=w54) -> ("TDC"=w47:sgl)  [unwired: 10 in]
      n312 = call "TDC_Selection.vi"("TDC#"=w53) -> ("TDC"=w46:sgl)  [unwired: 10 in]
      n313 = call "TDC_Selection.vi"("TDC#"=w52) -> ("TDC"=w45:sgl)  [unwired: 10 in]
      n314 = call "TDC_Selection.vi"("TDC#"=w51) -> ("TDC"=w44:sgl)  [unwired: 10 in]
      n315 = Bundle By Name(cluster=T3 {"MaxCAD"=0.0, "EPT Sim Enabled"=FALSE, "EPTxData"={"Sync"=FALSE, "CurrentCAD"=0.0, "Speed [RPM]"=0.0, "Config"=FALSE, "Rcvg Primary"=FALSE, "Stall"=FALSE, "Overflow"=FALSE, "Ratio Error"=FALSE, "Pattern Error"=FALSE, "Aux Warning"=FALSE, "Watchdog Error"=FALSE}} ("EPT in"), "EPTxData"=w85, "MaxCAD"=w88, "EPT Sim Enabled"=w119) -> (→"EPT out":T3)
      n316 = call "Hardware|EPTx|EncoderA"() -> ("Value"=w97:u8)
      n317 = call "Hardware|EPTx|EncoderB"() -> ("Value"=w96:u8)
      n318 = call "Hardware|EPTx|EncoderZ"() -> ("Value"=w95:u8)
      n319 = call "Hardware|EPTx|GateReset"() -> ("Value"=w94:u8)
      n320 = call "Hardware|EPTx|EncSignalSelect"() -> ("Value"=w93:bool)
      n321 = global write "TDC Globals.vi" "ESTTL2-1_TDC"(w43) -> ()
      n322 = global write "TDC Globals.vi" "ESTTL2-2_TDC"(w50) -> ()
      n323 = global write "TDC Globals.vi" "ESTTL2-3_TDC"(w49) -> ()
      n324 = global write "TDC Globals.vi" "ESTTL2-4_TDC"(w48) -> ()
      n325 = global write "TDC Globals.vi" "ESTTL2-5_TDC"(w47) -> ()
      n326 = global write "TDC Globals.vi" "ESTTL2-6_TDC"(w46) -> ()
      n327 = global write "TDC Globals.vi" "ESTTL2-7_TDC"(w45) -> ()
      n328 = global write "TDC Globals.vi" "ESTTL2-8_TDC"(w44) -> ()
      n329 = call "Hardware|EPTx|EngineStatus"("Value"=w79) -> ()
      n330 = call "Hardware|EPTx|PrimaryIndex"() -> ("Value"=w106:u8)
      n331 = call "Hardware|EPTx|Aux1Index"() -> ("Value"=w105:u8)
      n332 = call "Hardware|EPTx|Aux2Index"() -> ("Value"=w104:u8)
      n333 = call "Hardware|EPTx|Aux3Index"() -> ("Value"=w103:u8)
      n334 = call "Hardware|EPTx|Aux4Index"() -> ("Value"=w102:u8)
      n335 = disable-structure shown="CAS==TRUE" {
        disable-tunnel: w98 -> [w288 _]
        disable-tunnel: w97 -> [w287 _]
        disable-tunnel: w96 -> [w286 _]
        disable-tunnel: w95 -> [w285 _]
        disable-tunnel: w94 -> [w284 _]
        disable-tunnel: w93 -> [w283 _]
        disable-tunnel: w64 -> [w282 _]
        frame condition #0 (active) {
          n336 = xnode "Read/Write Control"("FPGA VI Reference In"=w288, "EPTxEncoderConfig"=w282, "EPTx.EncoderA"=w287, "EPTx.EncoderB"=w286, "EPTx.EncoderZ"=w285, "EPTx.Gate/Reset"=w284, "EPTx.EncSignalSelect"=w283) -> ()  [unwired: 1 in, 2 out]
        }
        frame condition #1 {
        }
      }
      n337 = xnode "Read/Write Control"("FPGA VI Reference In"=w98, "EPTx.Primary"=w106, "EPTx.Aux1"=w105, "EPTx.Aux2"=w104, "EPTx.Aux3"=w103, "EPTx.Aux4"=w102) -> ()  [unwired: 1 in, 2 out]
    }
    frame Error {
    }
  }
  n338 = call "Hardware|EPTx|FPGA1Error"("Value"=w10) -> ()
  n339 = call "Critical|EPTx|FPGA1Error"("Fault"=w10) -> ()  [unwired: 2 in]
